vi "Generating Integer LabVIEW Code.vi"() -> ()   [LabVIEW 2023]
uses:
  <vilib>/addons/Digital Filter Design/_Objects.llb/DFD Coef Norm Type.ctl
  <vilib>/addons/Digital Filter Design/FXPModel.llb/DFD FXP Quantize Coef (Easy).vi
  <vilib>/addons/Digital Filter Design/CodeGen.llb/DFD FXP Integer LabVIEW Code Generator.vi
  <vilib>/addons/Digital Filter Design/Process.llb/DFD Filtering (Array).vi
  <vilib>/Utility/VariantDataType/GetNumericFxpInfo.vi
  <vilib>/addons/Digital Filter Design/FXPSim.llb/dfd_Check Input FXP Settings.vi
  <vilib>/addons/Digital Filter Design/FXPSim.llb/dfd_Check SRate Simulation Integer Input.vi
  <vilib>/addons/Digital Filter Design/FXPSim.llb/dfd_FXP Simu.vi
  <vilib>/addons/Digital Filter Design/_Objects.llb/DFD Quantization Sources.ctl
  <vilib>/addons/Digital Filter Design/_Objects.llb/DFD FXP Statistics Data.ctl
  <vilib>/addons/Digital Filter Design/FXPSim.llb/SimXnode/DFD FXP Simulation.xnode
  <vilib>/addons/Digital Filter Design/_Objects.llb/DFD Filter Obj.ctl
  <vilib>/addons/Digital Filter Design/_Objects.llb/DFD Filter Coef.ctl
  <vilib>/addons/Digital Filter Design/_Objects.llb/DFD Filter Structure Type Selector.ctl
  <vilib>/addons/Digital Filter Design/_Objects.llb/dfd_Internal Quantization Settings.ctl
  <vilib>/addons/Digital Filter Design/_Objects.llb/dfd_Internal Quantization Srcs.ctl
  <vilib>/addons/Digital Filter Design/NI_DigFilterLicensed.lvlib
  <vilib>/addons/Digital Filter Design/NI_DigFilter_FXP.lvlib
  <vilib>/Utility/VariantDataType/VariantType.lvlib
panel:
  out "lvproj path":path
  in  "filter name":string
  in  "destination folder":path
  out "filtering text report":string
  out "Waveform Graph":dbl[][](graph)
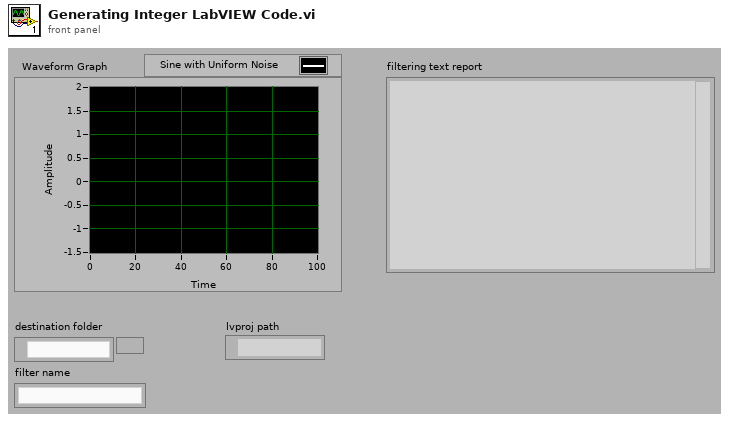
[diagram p1: front panel]
types:
  T1 = cluster{"gain processing":u16, "gain word length":i16}
  T2 = typedef "NI_DigFilterLicensed.lvlib/DFD Coef Norm Type.ctl" = enum16{"No Norm", "Time Domain 1-Norm", "Time Domain 2-Norm", "Time Domain Inf-Norm"}
  T3 = typedef "NI_DigFilterLicensed.lvlib/DFD Filter Obj.ctl" = cluster{"mSRate_Fs":dbl, "mSRate_Version":string, "mSRate_Comments":string, "mSRate_OrgCoef":T4, "mSRate_CurCoef":T4, "mSRate_Quantized?":bool, "mSRate_QCoef":T4, "mSRate_QSettings":T6[], "mSRate_Order":i32, "mSRate_Scaling":cluster{"mSRate_ScaleByPowerOf2?":bool, "mSRate_ScaleType":T2}}
  T4 = typedef "NI_DigFilterLicensed.lvlib/DFD Filter Coef.ctl" = cluster{"type":T5, "gain":dbl, "coef a (k)":dbl[], "coef b (v)":dbl[]}
  T5 = typedef "NI_DigFilterLicensed.lvlib/DFD Filter Structure Type Selector.ctl" = enum16{"Undefined", "FIR Direct Form", "FIR Direct Form Transposed", "FIR Symmetric", "FIR Antisymmetric", "IIR Direct Form I", "IIR Direct Form I Transposed", "IIR Direct Form II", "IIR Direct Form II Transposed", "IIR Cascaded Second Order Sections Form I", "IIR Cascaded Second Order Sections Form I Transposed", "IIR Cascaded Second Order Sections Form II", "IIR Cascaded Second Order Sections Form II Transposed", "Lattice Allpass (basic sections)", "Lattice Allpass (one multiplier sections)", "Lattice Allpass (normalized sections)", "Lattice AR (basic sections)", "Lattice AR (one multiplier sections)", "Lattice AR (normalized sections)", "Lattice MA (minimum phase)", "Lattice MA (maximum phase)", "Lattice ARMA (basic sections)", "Lattice ARMA (one multiplier sections)", "Lattice ARMA (normalized sections)"}
  T6 = typedef "NI_DigFilterLicensed.lvlib/dfd_Internal Quantization Settings.ctl" = cluster{"source":T7, "wl":i16, "iwl":i16, "overflow mode":enum16{"Saturation", "Wrap"}, "rounding mode":enum16{"Nearest", "Truncation"}, "signed?":bool}
  T7 = typedef "NI_DigFilterLicensed.lvlib/dfd_Internal Quantization Srcs.ctl" = u16
  T8 = typedef "NI_DigFilterLicensed.lvlib/DFD Quantization Sources.ctl" = u16
  T9 = typedef "NI_DigFilterLicensed.lvlib/DFD FXP Statistics Data.ctl" = cluster{"max value":ext, "min value":ext, "#overflows":i32, "#underflows":i32, "#operations":i32}
  T10 = cluster{"quantizer source":T8, "statistics information":T9}[]
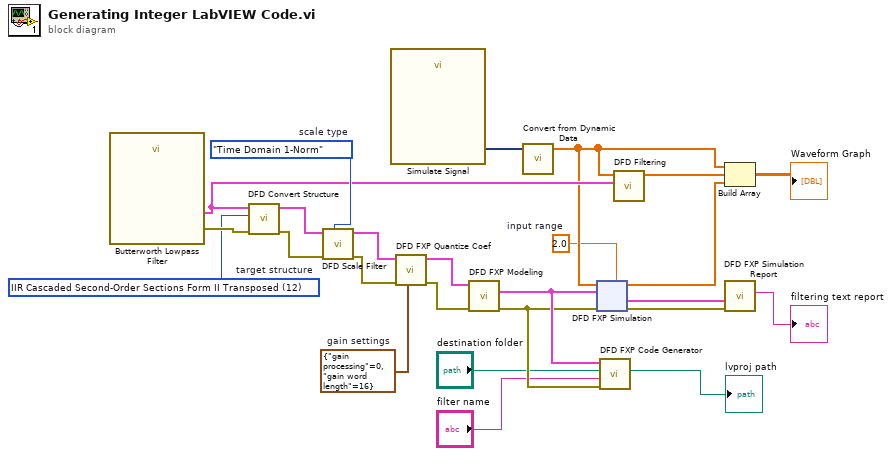
[diagram p0: block diagram]
diagram:
  w6 = 2.0  # input range
  w18 = T1 {"gain processing"=0, "gain word length"=16}  # gain settings
  w21 = DFD_Coef_Norm_Type."Time Domain 1-Norm"  # scale type
  w24 = u16 12 items=["FIR Direct Form"=1, "FIR Direct Form Transposed"=2, "FIR Symmetric"=3, "FIR Antisymmetric"=4, "IIR Direct Form I"=5, "IIR Direct Form I Transposed"=6, "IIR Direct Form II"=7, "IIR Direct Form II Transposed"=8, "IIR Cascaded Second-Order Sections Form I"=9, "IIR Cascaded Second-Order Sections Form I Transposed"=10, "IIR Cascaded Second-Order Sections Form II"=11, "IIR Cascaded Second-Order Sections Form II Transposed"=12, "Lattice Allpass (basic sections)"=13, "Lattice Allpass (one multiplier sections)"=14, "Lattice Allpass (normalized sections)"=15, "Lattice AR (basic sections)"=16, "Lattice AR (one multiplier sections)"=17, "Lattice AR (normalized sections)"=18, "Lattice MA (minimum phase)"=19, "Lattice MA (maximum phase)"=20, "Lattice ARMA (basic sections)"=21, "Lattice ARMA (one multiplier sections)"=22, "Lattice ARMA (normalized sections)"=23]  # target structure
  n1 = call "Butterworth Lowpass Filter"() -> ("error out"=w25:errorcluster, "filter out"=w14:T3)  [unwired: 1 in, 9 out]
  n2 = call <vilib>:"DFD Convert Structure.vi"("error in (no error)"=w25, "target structure"=w24, "filter in"=w14) -> ("error out"=w22:errorcluster, "filter out"=w23:T3)  [unwired: 7 out]
  n3 = call <vilib>:"DFD Scale Filter.vi"("scale type"=w21, "error in (no error)"=w22, "filter in"=w23) -> ("error out"=w19:errorcluster, "filter out"=w20:T3)  [unwired: 7 out]
  n4 = call "Simulate Signal"() -> ("Sine with Gaussian Noise"=w15:dynamicdata)  [unwired: 8 in, 7 out]
  n5 = call-poly <vilib>:"DFD FXP Quantize Coef.vi"("gain settings"=w18, "error in (no error)"=w19, "filter in"=w20) -> ("error out"=w16:errorcluster, "filter out"=w17:T3)  [unwired: 2 in, 5 out]
  n6 = call <vilib>:"DFD FXP Modeling.vi"("error in (no error)"=w16, "filter in"=w17) -> ("error out"=w4:errorcluster, "filter out"=w5:T3)  [unwired: 5 in, 3 out]
  n7 = call "Convert from Dynamic Data"("Dynamic Data Type"=w15) -> ("Array"=w13:dbl[])  [unwired: 3 out]
  n8 = xnode "DFD FXP Simulation"("input range"=w6, "error in (no error)"=w4, "filter in"=w5, "signal in"=w13) -> ("error out"=w9:errorcluster, "filtering statistics report"=w8:T10, "DBL signal out"=w11:dbl[])  [unwired: 2 in, 1 out]
  n9 = call-poly <vilib>:"DFD FXP Code Generator.vi"("error in (no error)"=w4, "filter name"="filter name", "destination folder"="destination folder", "filter in"=w5) -> ("lvproj path"=→"lvproj path":path)  [unwired: 3 in, 4 out]
  n10 = call-poly <vilib>:"DFD Filtering.vi"("filter"=w14, "signal in"=w13) -> ("signal out"=w12:dbl[])  [unwired: 2 in, 7 out]
  n11 = Build Array "Build Array"(w13, w12, w11) -> (→"Waveform Graph":dbl[][])
  n12 = call <vilib>:"DFD FXP Simulation Report.vi"("error in (no error)"=w9, "filtering statistics report"=w8) -> ("filtering text report"=→"filtering text report":string)  [unwired: 9 out]
